vi "Terminal.vi"() -> ()   [LabVIEW 2018, in "AlphaStep One.lvclass"]
uses:
  AlphaStep One.lvclass
  AlphaStep One.lvclass/AlphaStep One.ctl
  Serial Device/Serial Device.lvclass
panel:
  in  "Terminal":string
  out "RX Data":string
  out "AlphaStep One out":refnum<class "AlphaStep One.lvclass">
  in  "AlphaStep One in":refnum<class "AlphaStep One.lvclass">
  out "Error":errorcluster
  in  "Error In":errorcluster
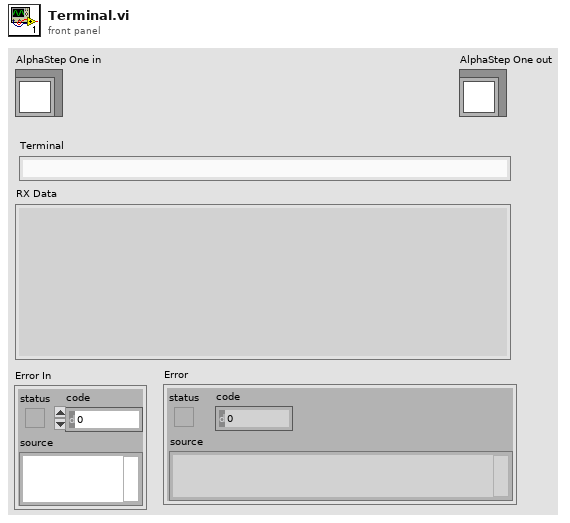
[diagram p1: front panel]
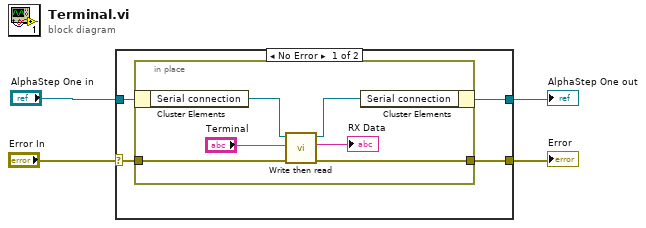
[diagram p0: block diagram]
diagram:
  n1 = case shown="No Error" "Error In" {
    selector: "Error In" -> [w7 w16]
    tunnel: [w6 w16] -> w3
    tunnel: "AlphaStep One in" -> [w5 w15]
    tunnel: [w8 w15] -> w1
    frame No Error {
      n2 = in-place {
        in-place-border: w7 -> [w13]
        in-place-border: [w12] -> w6
        n3 = in-place-cluster #1(w5) -> ("Serial connection"=w11:refnum<class "Serial Device.lvclass">)
        n4 = call "Write then read.vi"("error in (no error)"=w13, "TX Data"="Terminal", "Serial Device in"=w11) -> ("error out"=w12:errorcluster, "RX Data"=→"RX Data":string, "Serial Device out"=w14:refnum<class "Serial Device.lvclass">)  [unwired: 6 in]
        n5 = in-place-cluster #1("Serial connection"=w14) -> (w8:refnum<class "AlphaStep One.lvclass">)
      }
    }
    frame Error {
    }
  }
  "Error" <- w3
  "AlphaStep One out" <- w1
